vi "Frequency Components.vi"() -> ()   [LabVIEW 2023]
doc: "This example shows how to estimate the parameters of exponentially damped sinusoids with the TSA Modal Parametric Modeling VI. The parameters include magnitudes, phases, damping factors, and frequencies.\n\n<b>Instructions:</b>\n1) Run this VI.\n2) Set frequencies of the simulated signal.\n3) Observe the detected frequencies."
uses:
  <vilib>/addons/Time Series Analysis/Modeling and Prediction.llb/TSA Modal Parametric Modeling (Waveform).vi
  <vilib>/measure/NI_MABase.lvlib
  <vilib>/addons/_Advanced Signal Processing/NI_AdvSigProcTSA.lvlib
panel:
  in  "Noise":dbl=0.1 min=0.0 step=0.1
  in  "stop":bool
  in  "Model order":i32=4
  in  "Method":u16(ring)=1 items=["Prony", "Matrix Pencil"]
  out "sin(2p*f1) + sin(2p*f2) + Gaussian Noise":waveform(dbl)(graph)
  out "Frequencies (Hz)":dbl[](array[numeric]) format="%.1f"
  out "Amplitudes":dbl[](array[numeric]) format="%.2f"
  out "Damping factors":dbl[](array[numeric]) format="%.2f"
  out "Phases (deg)":dbl[](array[numeric]) format="%.1f"
  in  "f2 (Hz)":dbl=130.0 format="%.0p"
  in  "f1 (Hz)":dbl=120.0 format="%.0p"
  # "Overview: Shows how to estimate the parameters of exponentially damped sinusoids with the TSA Modal Parametric Modeling VI. The parameters include magnitudes, phases, damping factors, and frequencies.\nRequirements: LabVIEW Full Development System, Advanced Signal Processing Toolkit\nInstructions: \n1. Run this VI.\n2. Set frequencies of the simulated signal.\n3. Observe the detected frequencies.\n4. Click Stop to stop the VI."
  # "Signal Simulation"
  # "Settings"
  # "Estimated Parameters"
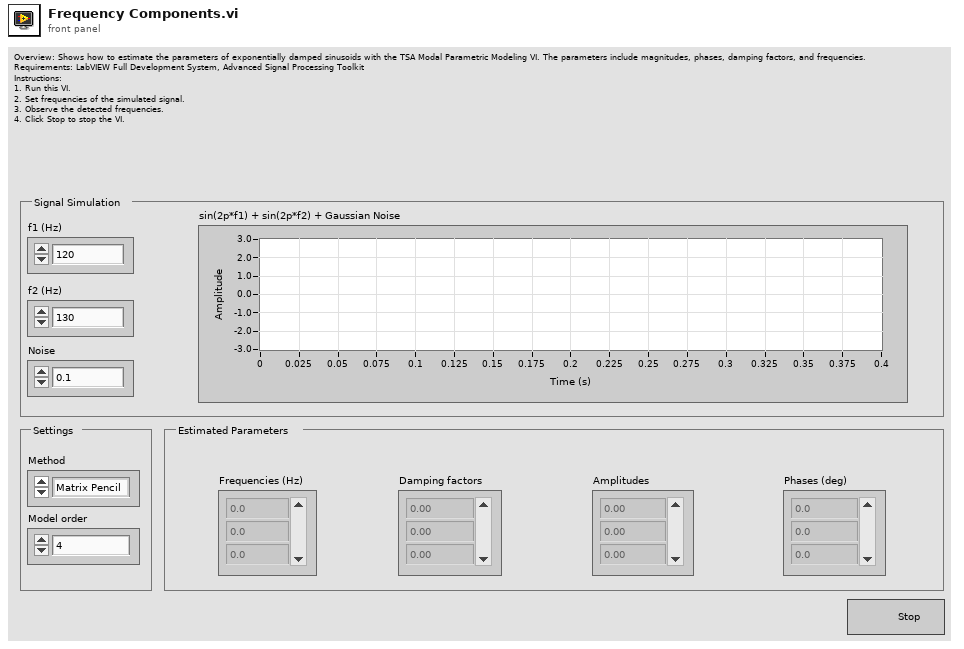
[diagram p1: front panel]
types:
  T1 = cluster{"frequency":dbl, "damping factor":dbl, "magnitude":dbl, "phase":dbl}[]
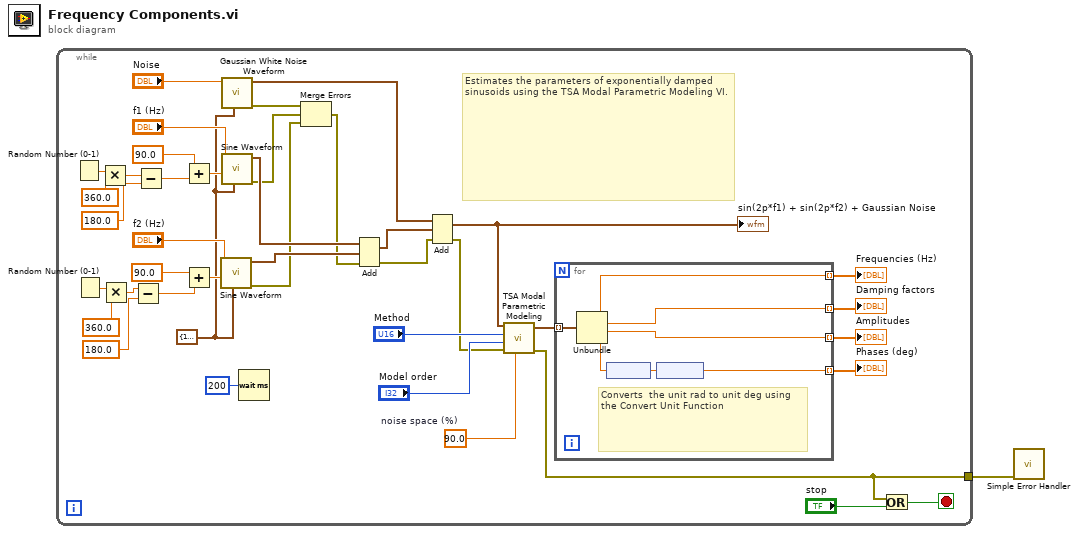
[diagram p0: block diagram]
diagram:
  n1 = while {
    tunnel: [w2] -> w1
    stop <- w15 stop-if-true
    w9 = 90.0  # noise space (%)
    w13 = cluster{"Fs":dbl, "#s":dbl} {"Fs"=1000.0, "#s"=400.0} ("Sampling Info")
    # "Estimates the parameters of exponentially damped sinusoids using the TSA Modal Parametric Modeling VI."
    n2 = Random Number (0-1)() -> (number: 0 to 1=w39:dbl)
    n3 = Random Number (0-1)() -> (number: 0 to 1=w37:dbl)
    n4 = Multiply(x=w39, y=360.0) -> (x*y=w34:dbl)
    n5 = Multiply(x=w37, y=360.0) -> (x*y=w32:dbl)
    n6 = Subtract(x=w32, y=180.0) -> (x-y=w25:dbl)
    n7 = Subtract(x=w34, y=180.0) -> (x-y=w35:dbl)
    n8 = Add(x=90.0, y=w35) -> (x+y=w42:dbl)
    n9 = Add(x=90.0, y=w25) -> (x+y=w41:dbl)
    n10 = call <vilib>:"Sine Waveform.vi"("sampling info"=w13, "phase"=w41, "frequency"="f2 (Hz)") -> ("error out"=w6:errorcluster, "signal out"=w19:waveform(dbl))  [unwired: 4 in, 3 out]
    n11 = call <vilib>:"Gaussian White Noise Waveform.vi"("sampling info"=w13, "standard deviation"="Noise") -> ("error out"=w8:errorcluster, "signal out"=w11:waveform(dbl))  [unwired: 3 in, 5 out]
    n12 = call <vilib>:"Sine Waveform.vi"("sampling info"=w13, "phase"=w42, "frequency"="f1 (Hz)") -> ("error out"=w7:errorcluster, "signal out"=w18:waveform(dbl))  [unwired: 4 in, 3 out]
    n13 = Wait (ms)(milliseconds to wait=u32 200 ("millisecond multiple")) -> ()  [unwired: 1 out]
    n14 = Merge Errors(w8, w7, w6) -> (w5:errorcluster)
    n15 = Add(1:w19, 2:w18, 4:w5) -> (0:w17:waveform(dbl), 3:w4:errorcluster)
    n16 = Add(1:w17, 2:w11, 4:w4) -> (0:w12:waveform(dbl), 3:w3:errorcluster)
    "sin(2p*f1) + sin(2p*f2) + Gaussian Noise" <- w12
    n17 = call-poly <vilib>:"TSA Modal Parametric Modeling.vi"("noise subspace (%)"=w9, "error in (no error)"=w3, "model order"="Model order", "method"="Method", "Xt"=w12) -> ("error out"=w2:errorcluster, "frequency components"=w30:T1)  [unwired: 5 out]
    n18 = for {
      tunnel: w30 -> [w48] mode=indexing
      tunnel: [w47] -> w29 mode=indexing
      tunnel: [w46] -> w28 mode=indexing
      tunnel: [w43] -> w27 mode=indexing
      tunnel: [w44] -> w26 mode=indexing
      # "Converts  the unit rad to unit deg using the Convert Unit Function"
      n19 = Unbundle(w48) -> ("frequency"=w47:dbl, "damping factor"=w46:dbl, "magnitude"=w43:dbl, "phase"=w45:dbl)
      n20 = node(w45) -> (w49:dbl[unit])
      n21 = node(w49) -> (w44:dbl)
    }
    "Phases (deg)" <- w26
    "Damping factors" <- w28
    "Amplitudes" <- w27
    "Frequencies (Hz)" <- w29
    n22 = Or(x=w2, y="stop") -> (x .or. y?=w15:bool)
  }
  n23 = call <vilib>:"Simple Error Handler.vi"("error in (no error)"=w1) -> ()  [unwired: 1 in, 8 out]
